vi "NaN_screening.vi"   [LabVIEW 2013]
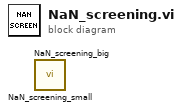
[diagram p0: block diagram]
diagram:
  n1 = call <userlib>:"NaN_screening_small.vi"() -> ()  [unwired: 11 in, 1 out]
  n2 = call <userlib>:"NaN_screening_big.vi"() -> ()  [unwired: 11 in, 1 out]
